vi "Initialise Low Poly Models.vi"(8 "error in (no error)":errorcluster, 10 "Number Of Objects":i32=10, 11 "Resource Directory":path) -> (0 "error out":errorcluster, 3 "Cubes":T1[](array[typedef]) {"Triangles"."Vertex 3"."UV"."v" min=0 max=1 step=0.1; "Triangles"."Vertex 3"."UV"."u" min=0 max=1 step=0.1; "Triangles"."Vertex 2"."UV"."v" min=0 max=1 step=0.1; "Triangles"."Vertex 2"."UV"."u" min=0 max=1 step=0.1; "Triangles"."Vertex 1"."UV"."v" min=0 max=1 step=0.1; "Triangles"."Vertex 1"."UV"."u" min=0 max=1 step=0.1})   [LabVIEW 2020, in "Scene.lvclass"]
uses:
  Scene.lvclass
  Scene.lvclass/Scene.ctl
  Graphics/Libraries/3D/3D.lvlib
  Graphics/Libraries/3D/Vector 3D.ctl
  Graphics/Libraries/3D/Transform.ctl
  <vilib>/numeric/Random Number (Range) DBL.vi
  <vilib>/numeric/Random Number (Range) I64.vi
  Graphics/Libraries/3D/Object.ctl
  Graphics/Libraries/Raster/UV.ctl
  Graphics/Libraries/Raster/Raster.lvlib
  Graphics/Libraries/3D/Vertex.ctl
  Graphics/Libraries/3D/Triangle.ctl
  Graphics/Libraries/Raster/Rectangle Dimensions.ctl
  Graphics/Libraries/Raster/Texture.ctl
  Graphics/Libraries/3D/Material.ctl
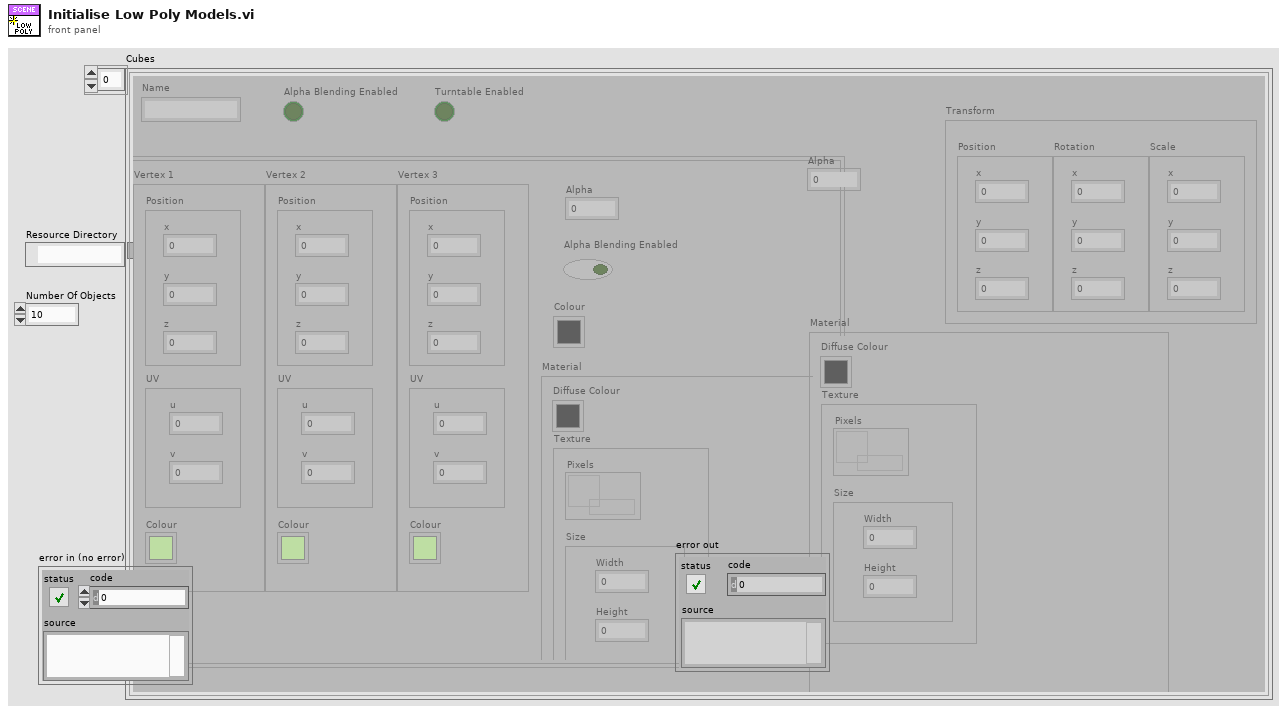
[diagram p1: front panel]
types:
  T1 = typedef "3D.lvlib/Object.ctl" = cluster{"Triangles":T2[], "Transform":T9, "Name":string, "Alpha Blending Enabled":bool, "Alpha":dbl, "Turntable Enabled":bool, "Material":T6}
  T2 = typedef "3D.lvlib/Triangle.ctl" = cluster{"Vertex 1":T3, "Vertex 2":T3, "Vertex 3":T3, "Alpha":dbl, "Alpha Blending Enabled":bool, "Colour":u32, "Material":T6}
  T3 = typedef "3D.lvlib/Vertex.ctl" = cluster{"Position":T4, "UV":T5, "Colour":u32}
  T4 = typedef "3D.lvlib/Vector 3D.ctl" = cluster{"x":sgl, "y":sgl, "z":sgl}
  T5 = typedef "Raster.lvlib/UV.ctl" = cluster{"u":sgl, "v":sgl}
  T6 = typedef "3D.lvlib/Material.ctl" = cluster{"Diffuse Colour":u32, "Texture":T7}
  T7 = typedef "Raster.lvlib/Texture.ctl" = cluster{"Pixels":refnum<data-value>, "Size":T8}
  T8 = typedef "Raster.lvlib/Rectangle Dimensions.ctl" = cluster{"Width":u32, "Height":u32}
  T9 = typedef "3D.lvlib/Transform.ctl" = cluster{"Position":T4, "Rotation":T4, "Scale":T4}
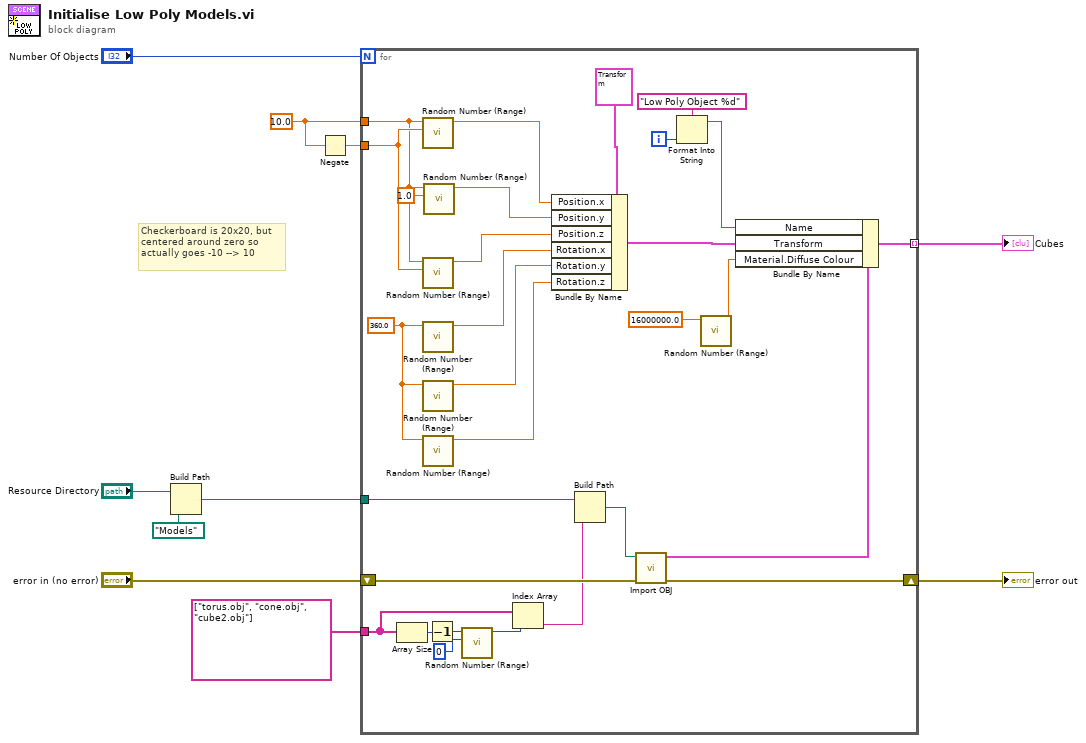
[diagram p0: block diagram]
diagram:
  w7 = 10.0 ("upper bound (100)")
  # "Checkerboard is 20x20, but centered around zero so actually goes -10 --> 10"
  n1 = Build Path(base path="Resource Directory", name or relative path=path "Models") -> (appended path=w2:path)
  n2 = Negate(x=w7) -> (-x=w6:dbl)
  n3 = for {
    N: "Number Of Objects" -> [_]
    tunnel: [w37] -> w8 mode=indexing
    tunnel: w7 -> [w12]
    tunnel: w6 -> [w31]
    shift-right: [w22] -> w3
    shift-left: "error in (no error)" -> [w24]
    tunnel: w2 -> [w21]
    tunnel: string[] ["torus.obj", "cone.obj", "cube2.obj"] -> [w19]
    i -> [w34]
    w27 = 360.0 ("upper bound (100)")
    n4 = Array Size(array=w19) -> (size(s)=w15:i32)
    n5 = call-poly <vilib>:"Random Number (Range).vi"("lower bound (0)"=w31, "upper bound (100)"=w12) -> ("number"=w33:dbl)  [unwired: 9 in]
    n6 = call-poly <vilib>:"Random Number (Range).vi"("lower bound (0)"=w31, "upper bound (100)"=w12) -> ("number"=w32:dbl)  [unwired: 9 in]
    n7 = call-poly <vilib>:"Random Number (Range).vi"("upper bound (100)"=w27) -> ("number"=w28:dbl)  [unwired: 10 in]
    n8 = call-poly <vilib>:"Random Number (Range).vi"("upper bound (100)"=w27) -> ("number"=w26:dbl)  [unwired: 10 in]
    n9 = call-poly <vilib>:"Random Number (Range).vi"("upper bound (100)"=w27) -> ("number"=w25:dbl)  [unwired: 10 in]
    n10 = call-poly <vilib>:"Random Number (Range).vi"("lower bound (0)"=1.0, "upper bound (100)"=w12) -> ("number"=w13:dbl)  [unwired: 9 in]
    n11 = Decrement(x=w15) -> (x-1=w14:i32)
    n12 = call-poly <vilib>:"Random Number (Range).vi"("lower bound (-100)"=i64 0, "upper bound (100)"=w14) -> ("number"=w18:i64)  [unwired: 9 in]
    n13 = Index Array(array=w19, index=w18) -> (element=w17:string)
    n14 = Bundle By Name(cluster=T9 {"Position"={"x"=2.0, "y"=1.0, "z"=-5.0}, "Rotation"={"x"=0.0, "y"=0.0, "z"=0.0}, "Scale"={"x"=0.0, "y"=0.0, "z"=0.0}} ("Transform"), "Position.x"=w33, "Position.y"=w13, "Position.z"=w32, "Rotation.x"=w28, "Rotation.y"=w26, "Rotation.z"=w25) -> (w38:T9)
    n15 = Build Path(base path=w21, name or relative path=w17) -> (appended path=w16:path)
    n16 = call "Import OBJ.vi"("error in (no error)"=w24, "Object"=w16) -> ("error out"=w22:errorcluster, "Object"=w23:T1)  [unwired: 8 in]
    n17 = Format Into String(format string="Low Poly Object %d" ("Name"), w34) -> (resulting string=w35:string)  [unwired: 2 in, 1 out]
    n18 = call-poly <vilib>:"Random Number (Range).vi"("upper bound (100)"=16000000.0) -> ("number"=w29:dbl)  [unwired: 10 in]
    n19 = Bundle By Name(cluster=w23, "Name"=w35, "Transform"=w38, "Material.Diffuse Colour"=w29) -> (w37:T1)
  }
  "Cubes" <- w8
  "error out" <- w3
